vi "Create.vi"(8 "error in (no error)":errorcluster) -> (0 "error out":errorcluster, 3 "Test Interface Mock Out":refnum<class "Test Interface Mock.lvclass">)   [LabVIEW 2020, in "Test Interface Mock.lvclass"]
uses:
  Test Interface Mock/Test Interface Mock.lvclass
  C:/git/astemes-lmock/sandbox/Mock/Mock.lvclass
  Mock/Mock.lvclass
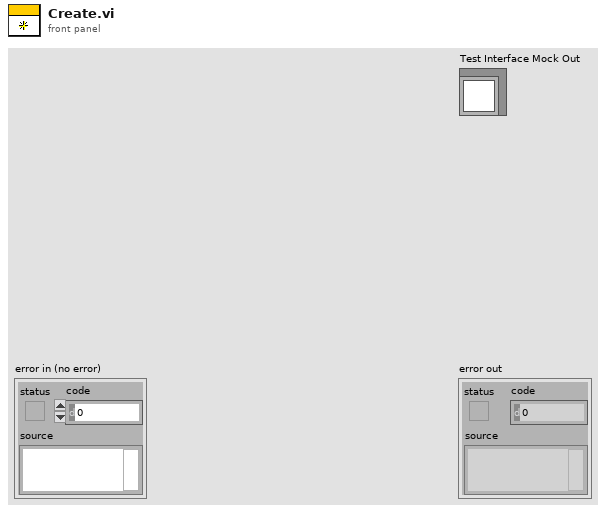
[diagram p1: front panel]
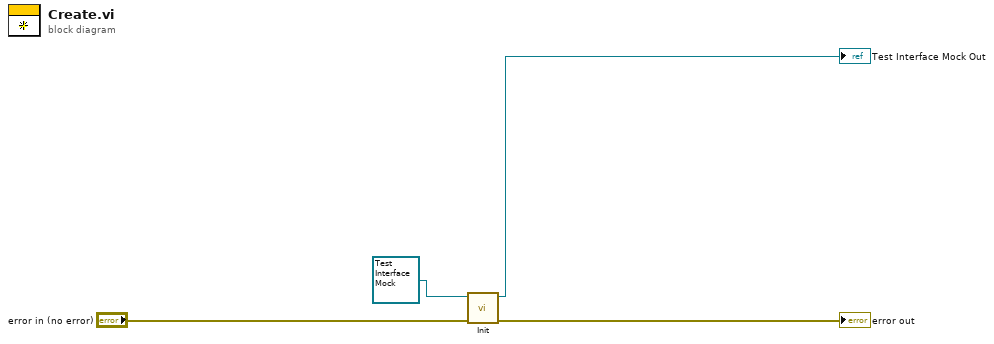
[diagram p0: block diagram]
diagram:
  n1 = call "Init.vi"("error in (no error)"="error in (no error)", "Mock in"=refnum<class "Test Interface Mock.lvclass"> refnum ("Test Interface Mock.lvclass")) -> ("error out"=→"error out":errorcluster, "Mock Out"=→"Test Interface Mock Out":refnum<class "Test Interface Mock.lvclass">)  [unwired: 8 in]
